vi "Vision Processing.vi"() -> ()   [LabVIEW 2016]
doc: "This VI runs in parallel to other tasks. It gets images from the camera, processes them for color or shape and use that information to affect robot behavior."
uses:
  <vilib>/Analysis/baseanly.llb/Mean (DBL).vi
  <vilib>/Instr/_visa.llb/VISA Configure Serial Port (Instr).vi
  <vilib>/Analysis/NI_AALBase.lvlib
panel:
  out "read buffer":string
  in  "VISA resource name":refnum<visa-resource-name>
  out "error out":errorcluster
  out "buffer":string
  in  "stop":bool
  out "error out 2":errorcluster
  out "X":i32
  out "Y":i32
  out "Width":i32
  out "Height":i32
  out "Area":dbl(graph)
  in  "Combo Box":string(combo)
  in  "Write":bool
  out "concatenated string":string
  in  "Flush":bool
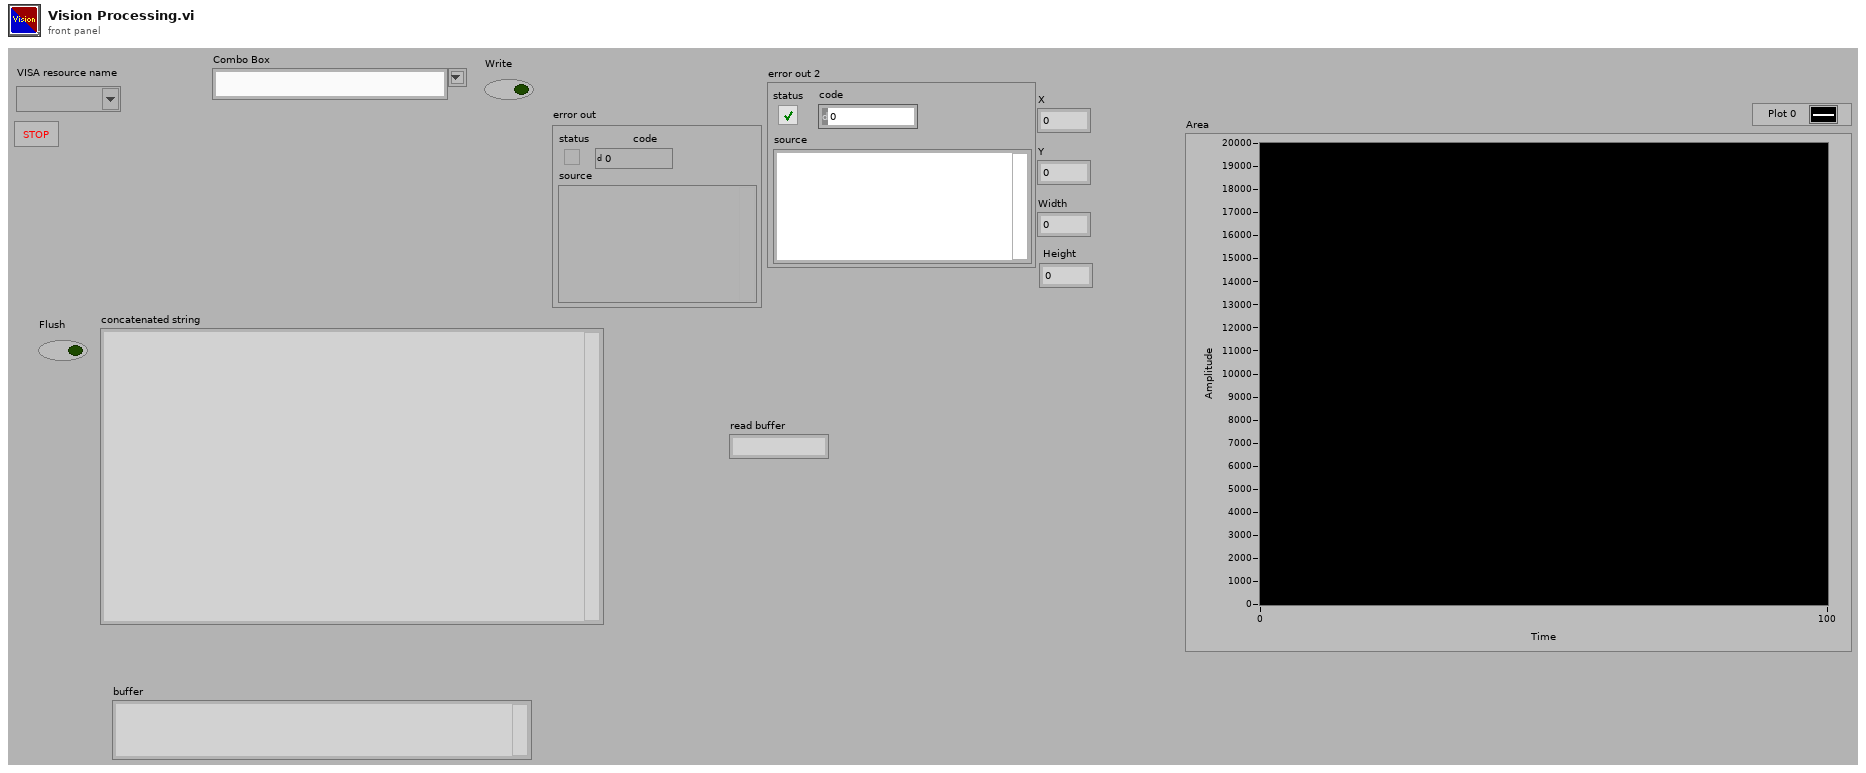
[diagram p1: front panel]
types:
  T1 = cluster{"buffer":string, "X":i32, "Y":i32, "Width":i32, "Height":i32, "Area":dbl}
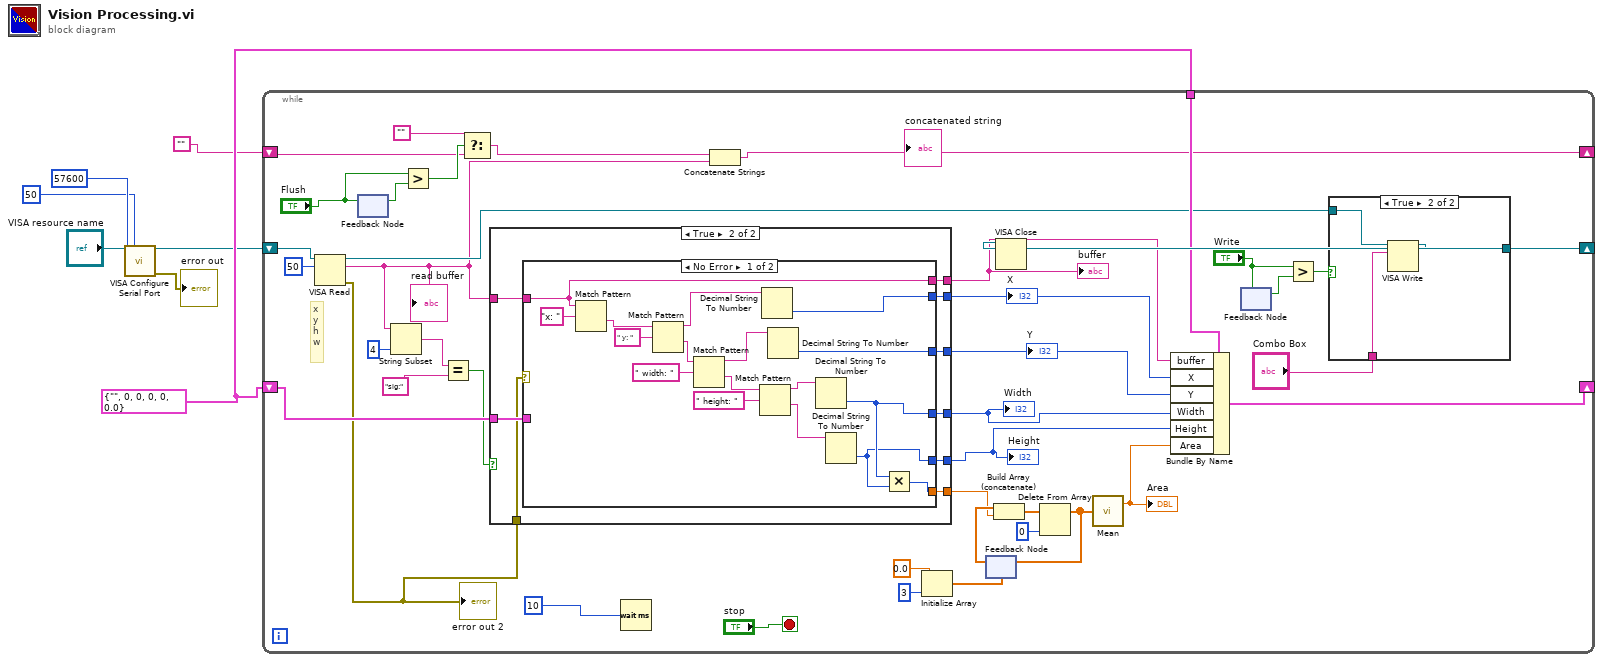
[diagram p0: block diagram]
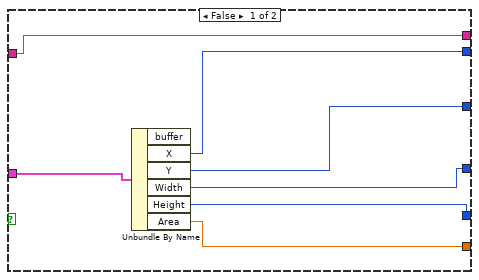
[diagram p2: hidden frame]
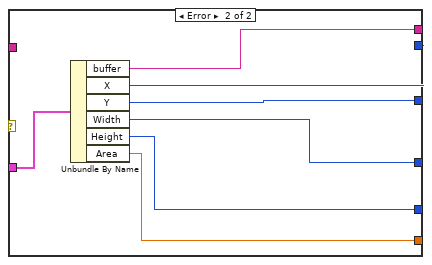
[diagram p3: hidden frame]
diagram:
  w3 = T1 {"buffer"="", "X"=0, "Y"=0, "Width"=0, "Height"=0, "Area"=0.0}
  n1 = call-poly "VISA Configure Serial Port"("VISA resource name"="VISA resource name", "timeout (10sec)"=u32 50, "baud rate (9600)"=u32 57600) -> ("VISA resource name out"=w1:refnum<visa-resource-name>, "error out"=→"error out":errorcluster)  [unwired: 11 in]
  n2 = while {
    shift-right: [w33] -> w8
    shift-left: w1 -> [w45]
    shift-right: [w44] -> _
    shift-left: w3 -> [w26]
    tunnel: w3 -> [w43]
    shift-right: [w16] -> _
    shift-left: "" -> [w12]
    stop <- "stop" stop-if-true
    # "x\ny\nh\nw"
    n3 = VISA Read(VISA resource name=w45, byte count=u32 50) -> (VISA resource name out=w34:refnum<visa-resource-name>, read buffer=w9:string, error out=w21:errorcluster)  [unwired: 1 in, 1 out]
    "error out 2" <- w21
    "read buffer" <- w9
    n4 = feedback #1() -> (w15:bool)  [unwired: 1 in]
    n5 = feedback-in #1("Flush") -> ()
    n6 = String Subset(string=w9, length (rest)=4 ("length (rest)")) -> (substring=w22:string)  [unwired: 1 in]
    n7 = Greater?(x="Flush", y=w15) -> (0:w13:bool)
    n8 = Equal?(x=w22, y="sig:") -> (x = y?=w24:bool)
    n9 = Select(t="", s=w13, f=w12) -> (s? t:f=w10:string)
    n10 = case shown="True" w24 {
      tunnel: [w49 w64] -> w32
      tunnel: [w54 w63] -> w31
      tunnel: [w53 w62] -> w30
      tunnel: [w52 w61] -> w29
      tunnel: [w51 w60] -> w28
      tunnel: [w50 w59] -> w27
      tunnel: w9 -> [w49 w58]
      tunnel: w26 -> [w55 w57]
      tunnel: w21 -> [_ w56]
      frame False {
        n11 = Unbundle By Name(w55) -> ("X"=w54:i32, "Y"=w53:i32, "Width"=w52:i32, "Height"=w51:i32, "Area"=w50:dbl)  [unwired: 1 out]
      }
      frame True {
        n12 = case shown="No Error" w56 {
          tunnel: [w77 w83] -> w63
          tunnel: [w73 w84] -> w62
          tunnel: [w68 w85] -> w61
          tunnel: [w67 w86] -> w60
          tunnel: [w66 w87] -> w59
          tunnel: w57 -> [_ w88]
          tunnel: w58 -> [w65 _]
          tunnel: [w65 w82] -> w64
          frame No Error {
            n13 = Match Pattern(string=w65, regular expression="x: ") -> (after substring=w80:string)  [unwired: 1 in, 3 out]
            n14 = Match Pattern(string=w80, regular expression=" y: ") -> (before substring=w78:string, after substring=w76:string)  [unwired: 1 in, 2 out]
            n15 = Match Pattern(string=w76, regular expression=" width: ") -> (before substring=w74:string, after substring=w72:string)  [unwired: 1 in, 2 out]
            n16 = Match Pattern(string=w72, regular expression=" height: ") -> (before substring=w70:string, after substring=w69:string)  [unwired: 1 in, 2 out]
            n17 = Decimal String To Number(string=w78) -> (number=w77:i32)  [unwired: 2 in, 1 out]
            n18 = Decimal String To Number(string=w74) -> (number=w73:i32)  [unwired: 2 in, 1 out]
            n19 = Decimal String To Number(string=w70) -> (number=w68:i32)  [unwired: 2 in, 1 out]
            n20 = Decimal String To Number(string=w69) -> (number=w67:i32)  [unwired: 2 in, 1 out]
            n21 = Multiply(x=w68, y=w67) -> (x*y=w66:i32)
          }
          frame Error {
            n22 = Unbundle By Name(w88) -> ("buffer"=w82:string, "X"=w83:i32, "Y"=w84:i32, "Width"=w85:i32, "Height"=w86:i32, "Area"=w87:dbl)
          }
        }
      }
    }
    "buffer" <- w32
    "X" <- w31
    "Y" <- w30
    "Width" <- w29
    "Height" <- w28
    n23 = Wait (ms)(milliseconds to wait=u32 10) -> ()  [unwired: 1 out]
    n24 = Concatenate Strings(w10, w9) -> (w16:string)
    "concatenated string" <- w16
    n25 = Initialize Array(0.0 ("element"), 3 ("dimension size")) -> (w39:dbl[])
    n26 = feedback #2(w39) -> (w35:dbl[])
    n27 = Build Array (concatenate)(w35, w27) -> (w38:dbl[])
    n28 = Delete From Array(array=w38, index=0) -> (array with subset deleted=w37:dbl[])  [unwired: 1 in, 1 out]
    n29 = feedback-in #2(w37) -> ()
    n30 = call-poly <vilib>:"Mean.vi"("X"=w37) -> ("mean"=w42:dbl)  [unwired: 1 out]
    "Area" <- w42
    n31 = Bundle By Name(cluster=w43, "buffer"=w32, "X"=w31, "Y"=w30, "Width"=w29, "Height"=w28, "Area"=w42) -> (w44:T1)
    n32 = feedback-in #3("Write") -> ()
    n33 = feedback #3() -> (w18:bool)  [unwired: 1 in]
    n34 = Greater?(x="Write", y=w18) -> (0:w19:bool)
    n35 = case shown="True" w19 {
      tunnel: w34 -> [w89 w92]
      tunnel: [w89 w91] -> w33
      tunnel: "Combo Box" -> [_ w90]
      frame False {
      }
      frame True {
        n36 = VISA Write(VISA resource name=w92, write buffer=w90) -> (VISA resource name out=w91:refnum<visa-resource-name>)  [unwired: 1 in, 2 out]
      }
    }
  }
  n37 = VISA Close(VISA resource name=w8) -> ()  [unwired: 1 in, 1 out]
